vi "Cancel.vi"(9 "CancellationReason":errorcluster, 11 "JQMHStartup in":refnum<class "RQMHStartup.lvclass">) -> (0 "error out":errorcluster)   [LabVIEW 2024, in "RQMHStartup.lvclass"]
uses:
  RQMHStartup.lvclass
  Command.ctl
  RQMHStartup.lvclass/RQMHStartup.ctl
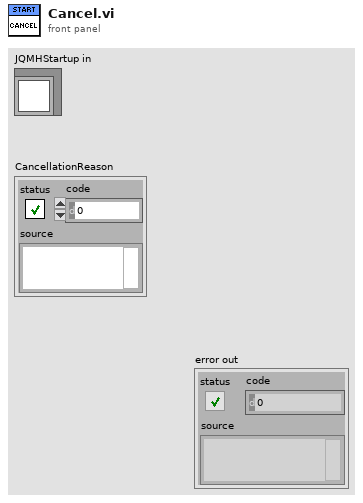
[diagram p1: front panel]
types:
  T1 = typedef "RQMHStartup.lvclass/Command.ctl" = enum16{"Default", "No Override", "Error", "ACK Created", "ACK Mod Reg", "ACK Caller Reg"}
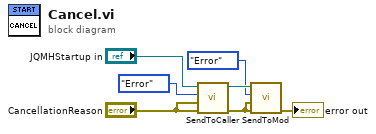
[diagram p0: block diagram]
diagram:
  n1 = call "SendToCaller.vi"("error in (no error)"="CancellationReason", "Data"="CancellationReason", "Command"=Command."Error", "JQMHStartup in"="JQMHStartup in") -> ("error out"=w1:errorcluster, "JQMHStartup out"=w5:refnum<class "RQMHStartup.lvclass">)  [unwired: 6 in]
  n2 = call "SendToMod.vi"("error in (no error)"=w1, "Data"=w1, "Command"=Command."Error", "JQMHStartup in"=w5) -> ("error out"=→"error out":errorcluster)  [unwired: 6 in, 1 out]
